vi "Show DBL postfix.vi"() -> ()   [LabVIEW 2017]
panel:
  out "Array 2":string[](array[string])
  out "Array":string[](array[string])
  out "resulting string":string
  in  "input 1":dbl format="%#_15p"
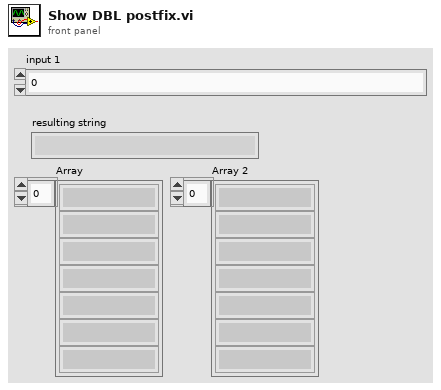
[diagram p1: front panel]
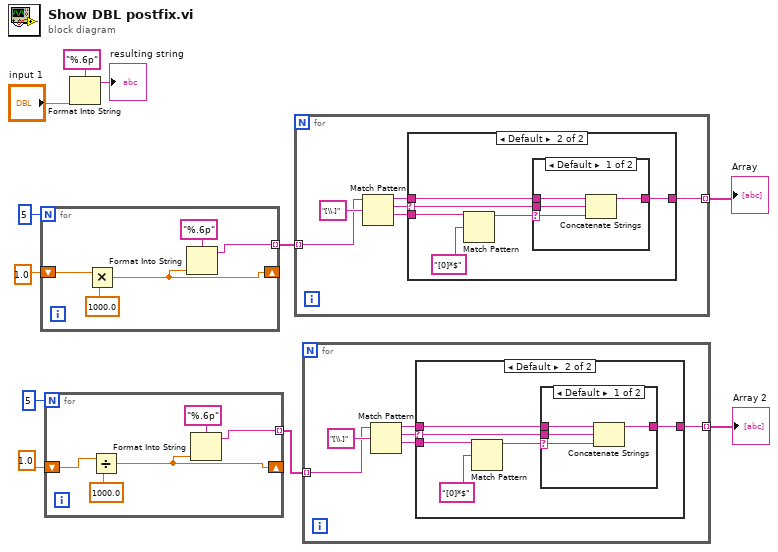
[diagram p0: block diagram]
diagram:
  n1 = for {
    N: 5 -> [_]
    shift-right: [w13] -> _
    shift-left: 1.0 ("input 2") -> [w16]
    tunnel: [w12] -> w4 mode=indexing
    n2 = Multiply(x=w16, y=1000.0) -> (x*y=w13:dbl)
    n3 = Format Into String(format string="%.6p", w13) -> (resulting string=w12:string)  [unwired: 2 in, 1 out]
  }
  n4 = for {
    N: 5 -> [_]
    shift-right: [w18] -> _
    shift-left: 1.0 ("input 2") -> [w21]
    tunnel: [w17] -> w2 mode=indexing
    n5 = Divide(x=w21, y=1000.0) -> (x/y=w18:dbl)
    n6 = Format Into String(format string="%.6p", w18) -> (resulting string=w17:string)  [unwired: 2 in, 1 out]
  }
  n7 = Format Into String(format string="%.6p", "input 1") -> (resulting string=→"resulting string":string)  [unwired: 2 in, 1 out]
  n8 = for {
    tunnel: w4 -> [w23] mode=indexing
    tunnel: [w22] -> w3 mode=indexing
    n9 = Match Pattern(string=w23, regular expression="[\\.]") -> (before substring=w25:string, match substring=w24:string, after substring=w26:string)  [unwired: 1 in, 1 out]
    n10 = case shown="Default" w24 {
      selector: w24 -> [_ w31]
      tunnel: w26 -> [_ w34]
      tunnel: w25 -> [w28 w32]
      tunnel: [w28 w29] -> w22
      frame "" {
      }
      frame Default {
        n11 = Match Pattern(string=w34, regular expression="[0]*$") -> (before substring=w30:string)  [unwired: 1 in, 3 out]
        n12 = case shown="Default" w30 {
          selector: w30 -> [w36 _]
          tunnel: w32 -> [w38 w39]
          tunnel: w31 -> [w37 _]
          tunnel: [w35 w39] -> w29
          frame Default {
            n13 = Concatenate Strings(w38, w37, w36) -> (w35:string)
          }
          frame "" {
          }
        }
      }
    }
  }
  "Array" <- w3
  n14 = for {
    tunnel: w2 -> [w41] mode=indexing
    tunnel: [w40] -> w1 mode=indexing
    n15 = Match Pattern(string=w41, regular expression="[\\.]") -> (before substring=w43:string, match substring=w42:string, after substring=w44:string)  [unwired: 1 in, 1 out]
    n16 = case shown="Default" w42 {
      selector: w42 -> [_ w49]
      tunnel: w44 -> [_ w52]
      tunnel: w43 -> [w46 w50]
      tunnel: [w46 w47] -> w40
      frame "" {
      }
      frame Default {
        n17 = Match Pattern(string=w52, regular expression="[0]*$") -> (before substring=w48:string)  [unwired: 1 in, 3 out]
        n18 = case shown="Default" w48 {
          selector: w48 -> [w54 _]
          tunnel: w50 -> [w56 w57]
          tunnel: w49 -> [w55 _]
          tunnel: [w53 w57] -> w47
          frame Default {
            n19 = Concatenate Strings(w56, w55, w54) -> (w53:string)
          }
          frame "" {
          }
        }
      }
    }
  }
  "Array 2" <- w1
